vi "Test Type Disables.vi"(2 "TestTypeControls[]":refnum<vi>[](array[refnum]), 5 "TestType":enum32{"Flow", "Timed", "Hot\nFuel"}(ring), 6 "table.Data":string[][](array[string])) -> ()   [LabVIEW 2013]
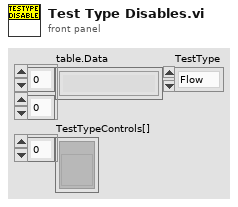
[diagram p1: front panel]
types:
  T1 = enum8{"Enabled", "Disabled", "Disabled and Grayed Out"}[]
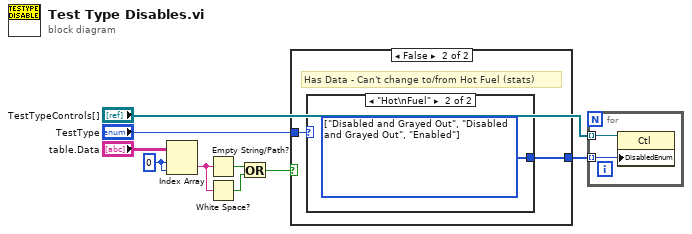
[diagram p0: block diagram]
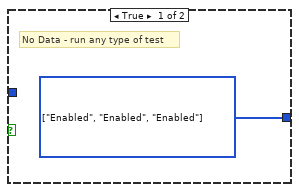
[diagram p2: hidden frame]
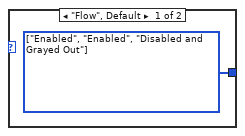
[diagram p3: hidden frame]
diagram:
  w7 = 0 ("index (row)")
  n1 = Index Array(array="table.Data", index (row)=w7, index (col)=w7) -> (element=w6:string)
  n2 = Empty String/Path?(string/path=w6) -> (empty?=w5:bool)
  n3 = White Space?(1:w6) -> (0:w4:bool)
  n4 = Or(x=w5, y=w4) -> (x .or. y?=w8:bool)
  n5 = case shown="False" w8 {
    tunnel: "TestType" -> [_ w12]
    tunnel: [w10 w11] -> w9
    frame True {
      w10 = T1 [enum."Enabled", enum."Enabled", enum."Enabled"] items=["Enabled", "Disabled", "Disabled and Grayed Out"]
      # "No Data - run any type of test"
    }
    frame False {
      # "Has Data - Can't change to/from Hot Fuel (stats)"
      n6 = case shown="\"Hot\\nFuel\"" w12 {
        tunnel: [w13 w14] -> w11
        frame "Flow", Default {
          w13 = T1 [enum."Enabled", enum."Enabled", enum."Disabled and Grayed Out"] items=["Enabled", "Disabled", "Disabled and Grayed Out"]
        }
        frame "Hot\nFuel" {
          w14 = T1 [enum."Disabled and Grayed Out", enum."Disabled and Grayed Out", enum."Enabled"] items=["Enabled", "Disabled", "Disabled and Grayed Out"]
        }
      }
    }
  }
  n7 = for {
    tunnel: "TestTypeControls[]" -> [w16] mode=indexing
    tunnel: w9 -> [w15] mode=indexing
    n8 = property class="Ctl"(reference=w16, "DisabledEnum"=w15) -> ()  [unwired: 1 in, 2 out]
  }
